vi "FileandHeader.vi"(0 "operation (0:open)":T1(ring), 1 "string":string, 4 "Specified sampling rate":dbl, 5 "Specified generated frequency (Hz)":dbl, 6 "reference":refnum<vi>, 8 "Device name":string, 9 "Gen sample rate":dbl, 11 "Read sample rate":dbl) -> (14 "write":refnum<file>, 15 "error out 2":errorcluster, 16 "airflow refnum out":refnum<file>, 17 "Airflow error":errorcluster, 18 "read":refnum<file>, 19 "error out":errorcluster)   [LabVIEW 2017]
panel:
  out "concatenated string":string
  # "© The Regents of the University of California, Davis campus, 2019. This material is available as open source for research and personal use under a Creative Commons Attribution-NonCommercial-NoDerivatives 4.0 International Public License (https://creativecommons.org/licenses/by-nc-nd/4.0/)."
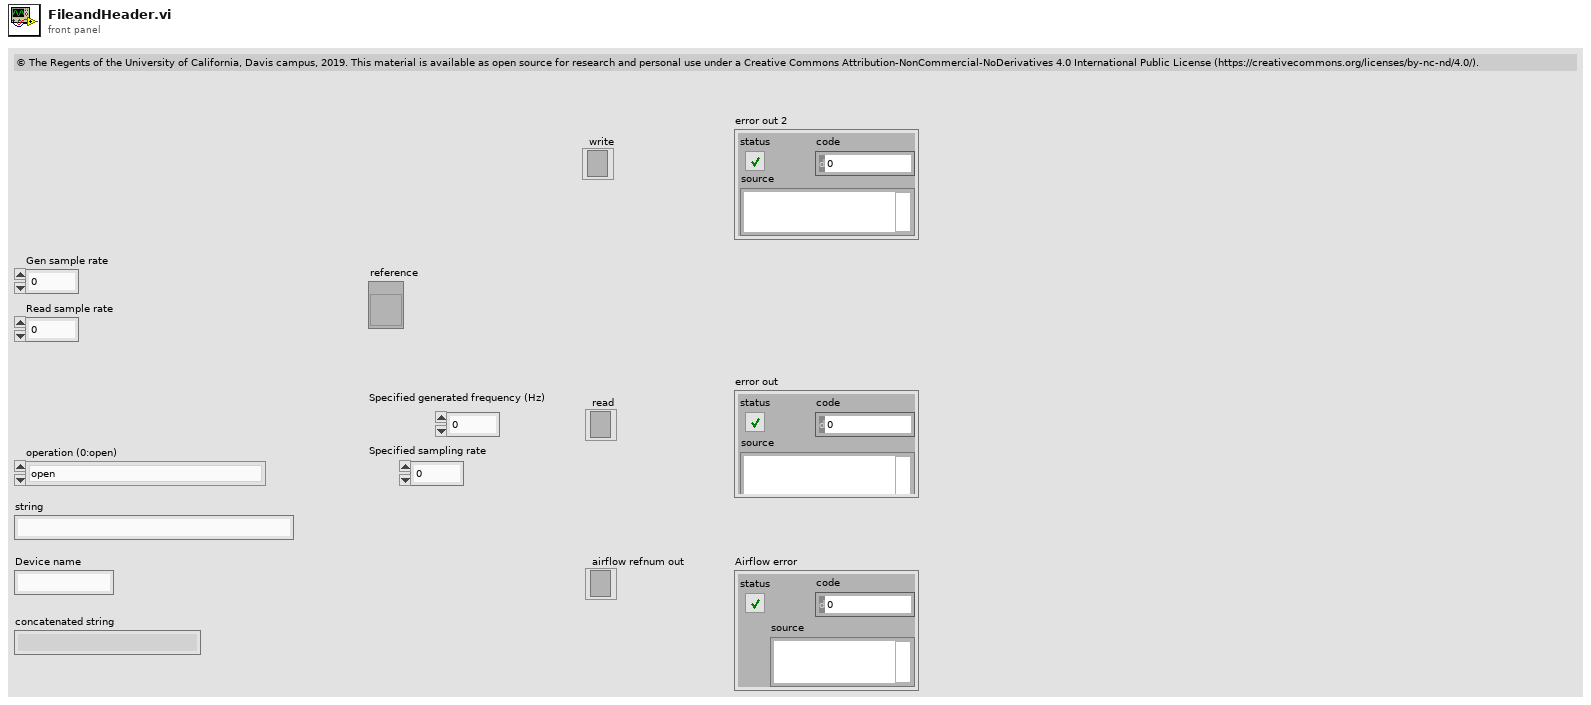
[diagram p1: front panel]
types:
  T1 = enum16{"open", "replace", "create", "open or create", "replace or create", "replace or create with confirmation"}
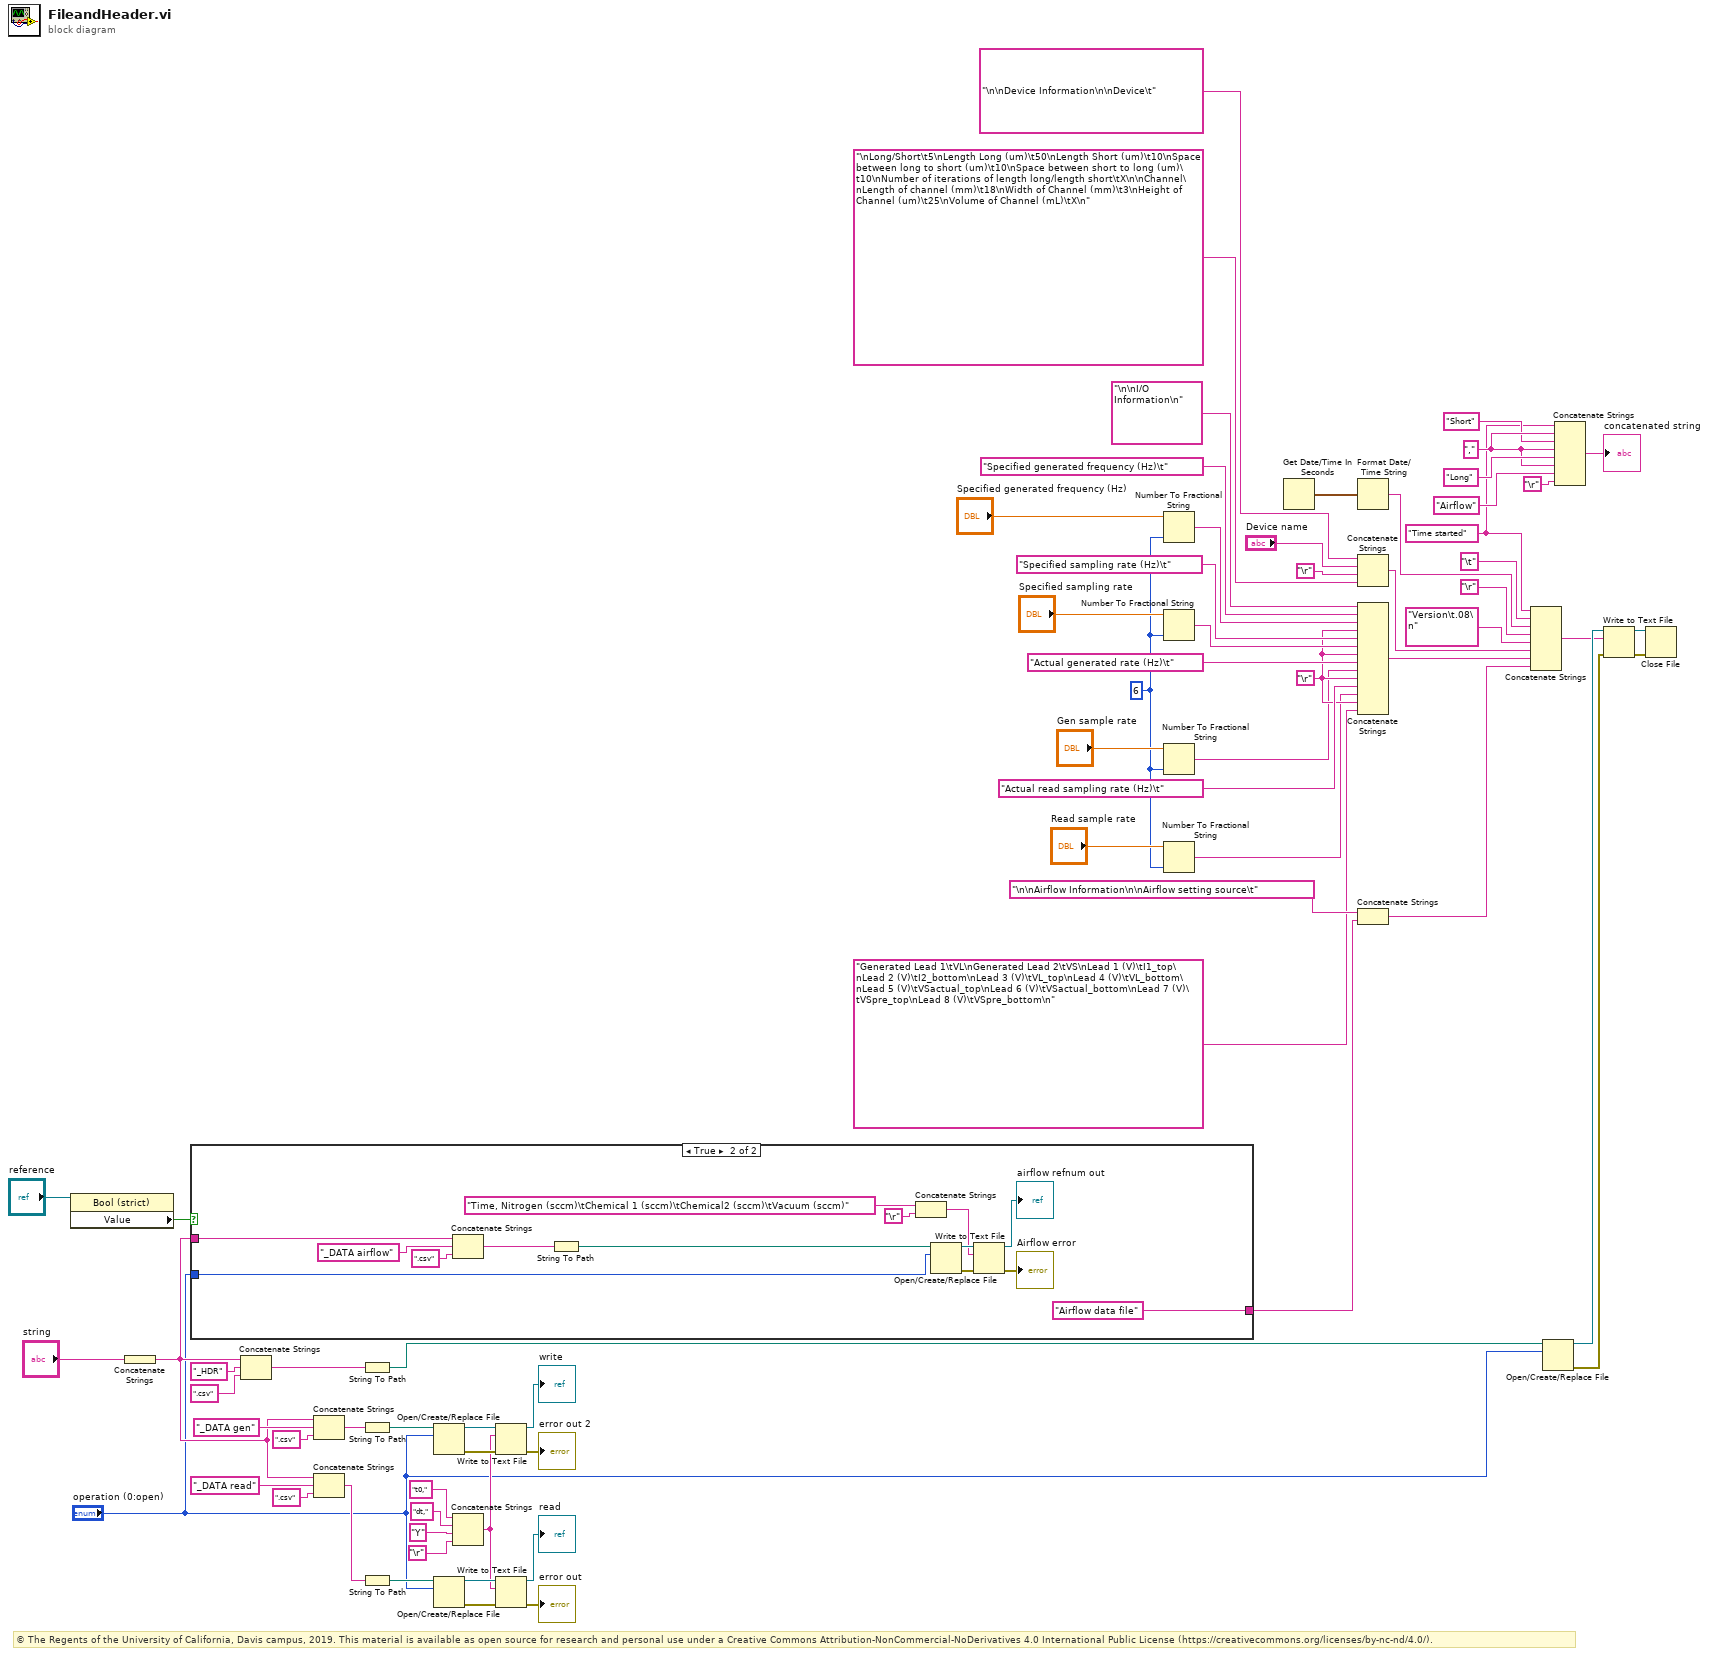
[diagram p0: block diagram]
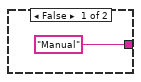
[diagram p2: hidden frame]
diagram:
  w13 = "\r"
  w53 = "," ("string")
  w2 = i16 6 ("width (-)")
  w49 = "Time started" ("string")
  # "© The Regents of the University of California, Davis campus, 2019. This material is available as open source for research and personal use under a Creative Commons Attribution-NonCommercial-NoDerivatives 4.0 International Public License (https://creativecommons.org/licenses/by-nc-nd/4.0/)."
  n1 = property on="Property Node" class="Bool (strict)"(reference="reference") -> ("Value"=w31:bool)  [unwired: 1 in, 2 out]
  n2 = Concatenate Strings("string") -> (w28:string)
  n3 = case shown="True" w31 {
    tunnel: ["Manual" ("string") "Airflow data file" ("string")] -> w24
    tunnel: w28 -> [_ w80]
    tunnel: "operation (0:open)" -> [_ w77]
    frame False {
    }
    frame True {
      n4 = Concatenate Strings(w80, "_DATA airflow" ("string"), ".csv" ("string")) -> (w82:string)
      n5 = String To Path(string=w82) -> (path=w78:path)
      n6 = Concatenate Strings("Time, Nitrogen (sccm)\tChemical 1 (sccm)\tChemical2 (sccm)\tVacuum (sccm)" ("text"), "\r") -> (w74:string)
      n7 = Open/Create/Replace File(file path (use dialog)=w78, operation (0:open)=w77) -> (refnum out=w86:refnum<file>, error out=w85:errorcluster)  [unwired: 4 in, 1 out]
      n8 = Write to Text File(file (use dialog)=w86, text=w74, error in=w85) -> (refnum out=→"airflow refnum out":refnum<file>, error out=→"Airflow error":errorcluster)  [unwired: 1 in, 1 out]
    }
  }
  n9 = Concatenate Strings(w28, "_HDR" ("string"), ".csv" ("string")) -> (w70:string)
  n10 = Concatenate Strings(w28, "_DATA gen" ("string"), ".csv" ("string")) -> (w57:string)
  n11 = Concatenate Strings(w28, "_DATA read" ("string"), ".csv" ("string")) -> (w62:string)
  n12 = String To Path(string=w70) -> (path=w69:path)
  n13 = String To Path(string=w57) -> (path=w37:path)
  n14 = String To Path(string=w62) -> (path=w38:path)
  n15 = Open/Create/Replace File(file path (use dialog)=w37, operation (0:open)="operation (0:open)") -> (refnum out=w47:refnum<file>, error out=w46:errorcluster)  [unwired: 4 in, 1 out]
  n16 = Open/Create/Replace File(file path (use dialog)=w38, operation (0:open)="operation (0:open)") -> (refnum out=w45:refnum<file>, error out=w44:errorcluster)  [unwired: 4 in, 1 out]
  n17 = Concatenate Strings("t0," ("string"), "dt," ("string"), "Y" ("string"), "\r") -> (w40:string)
  n18 = Write to Text File(file (use dialog)=w47, text=w40, error in=w46) -> (refnum out=→"write":refnum<file>, error out=→"error out 2":errorcluster)  [unwired: 1 in, 1 out]
  n19 = Write to Text File(file (use dialog)=w45, text=w40, error in=w44) -> (refnum out=→"read":refnum<file>, error out=→"error out":errorcluster)  [unwired: 1 in, 1 out]
  n20 = Number To Fractional String(number="Specified generated frequency (Hz)", precision (6)=w2) -> (F-format string=w18:string)  [unwired: 2 in]
  n21 = Number To Fractional String(number="Specified sampling rate", precision (6)=w2) -> (F-format string=w16:string)  [unwired: 2 in]
  n22 = Number To Fractional String(number="Gen sample rate", precision (6)=w2) -> (F-format string=w1:string)  [unwired: 2 in]
  n23 = Number To Fractional String(number="Read sample rate", precision (6)=w2) -> (F-format string=w4:string)  [unwired: 2 in]
  n24 = Get Date/Time In Seconds() -> (seconds since 1Jan1904=w68:timestamp)
  n25 = Format Date/Time String(seconds (now)=w68) -> (date/time string=w32:string)  [unwired: 2 in]
  n26 = Concatenate Strings("\n\nDevice Information\n\nDevice\t" ("string"), "Device name", "\r", "\nLong/Short\t5\nLength Long (um)\t50\nLength Short (um)\t10\nSpace between long to short (um)\t10\nSpace between short to long (um)\t10\nNumber of iterations of length long/length short\tX\n\nChannel\nLength of channel (mm)\t18\nWidth of Channel (mm)\t3\nHeight of Channel (um)\t25\nVolume of Channel (mL)\tX\n" ("string")) -> (w8:string)
  n27 = Concatenate Strings("\n\nI/O Information\n" ("string"), "Specified generated frequency (Hz)\t" ("string"), w18, w13, "Specified sampling rate (Hz)\t" ("string"), w16, w13, "Actual generated rate (Hz)\t" ("string"), w1, w13, "Actual read sampling rate (Hz)\t" ("string"), w4, w13, "Generated Lead 1\tVL\nGenerated Lead 2\tVS\nLead 1 (V)\tI1_top\nLead 2 (V)\tI2_bottom\nLead 3 (V)\tVL_top\nLead 4 (V)\tVL_bottom\nLead 5 (V)\tVSactual_top\nLead 6 (V)\tVSactual_bottom\nLead 7 (V)\tVSpre_top\nLead 8 (V)\tVSpre_bottom\n" ("string")) -> (w7:string)
  n28 = Concatenate Strings("\n\nAirflow Information\n\nAirflow setting source\t" ("string"), w24) -> (w6:string)
  n29 = Concatenate Strings(w49, "\t" ("string"), w32, "\r", "Version\t.08\n" ("string"), w8, w7, w6) -> (w65:string)
  n30 = Open/Create/Replace File(file path (use dialog)=w69, operation (0:open)="operation (0:open)") -> (refnum out=w67:refnum<file>, error out=w66:errorcluster)  [unwired: 4 in, 1 out]
  n31 = Concatenate Strings(w49, w53, "Short" ("string"), w53, "Long" ("string"), w53, "Airflow" ("string"), "\r") -> (→"concatenated string":string)
  n32 = Write to Text File(file (use dialog)=w67, text=w65, error in=w66) -> (refnum out=w64:refnum<file>, error out=w63:errorcluster)  [unwired: 1 in, 1 out]
  n33 = Close File(refnum=w64, error in=w63) -> ()  [unwired: 2 out]
